vi "Final_Project_Follower_Template-1.vi"   [LabVIEW 2016]
uses:
  <vilib>/NXT/Block Support/NXT_InputPort.ctl
  <vilib>/NXT/Block Support/NXT_TimerIndex.ctl
  <vilib>/NXT/Block Support/NXT_OutputPort.ctl
  <vilib>/NXT/Dual Mode Library/Sensors/EV3_Color_Reflect.vi
  <vilib>/NXT/Dual Mode Library/Display/drawText_Right.vi
  <vilib>/NXT/NXTIO Xnodes/NXTIONodeSubVIs/NXTStopMotors.vi
  <vilib>/NXT/Dual Mode Library/Sensors/EV3_Ultrasonic_CM.vi
  <vilib>/NXT/NXTIO Xnodes/NXTIONodeSubVIs/NXTMoveMotors.vi
  <vilib>/NXT/Dual Mode Library/Display/drawNumber.vi
  <vilib>/NXT/Dual Mode Library/Display/drawNumber_float.vi
  <vilib>/NXT/Dual Mode Library/Display/drawText.vi
  <vilib>/NXT/Subs/LVHSConnector.ctl
  <vilib>/NXT/NXTIO Xnodes/AddressXNode/NXTIOAddress.xnode
  <vilib>/NXT/NXTIO Xnodes/NXTIOXNode/NXTIO.xnode
  <vilib>/NXT/LegoClasses/BrickReference/BrickReference.lvclass
types:
  T1 = typedef "LVHSConnector.ctl" = refnum<class "BrickReference.lvclass">
  T2 = typedef "NXT_InputPort.ctl" = u32
  T3 = typedef "NXT_TimerIndex.ctl" = u8
  T4 = typedef "NXT_OutputPort.ctl" = u8
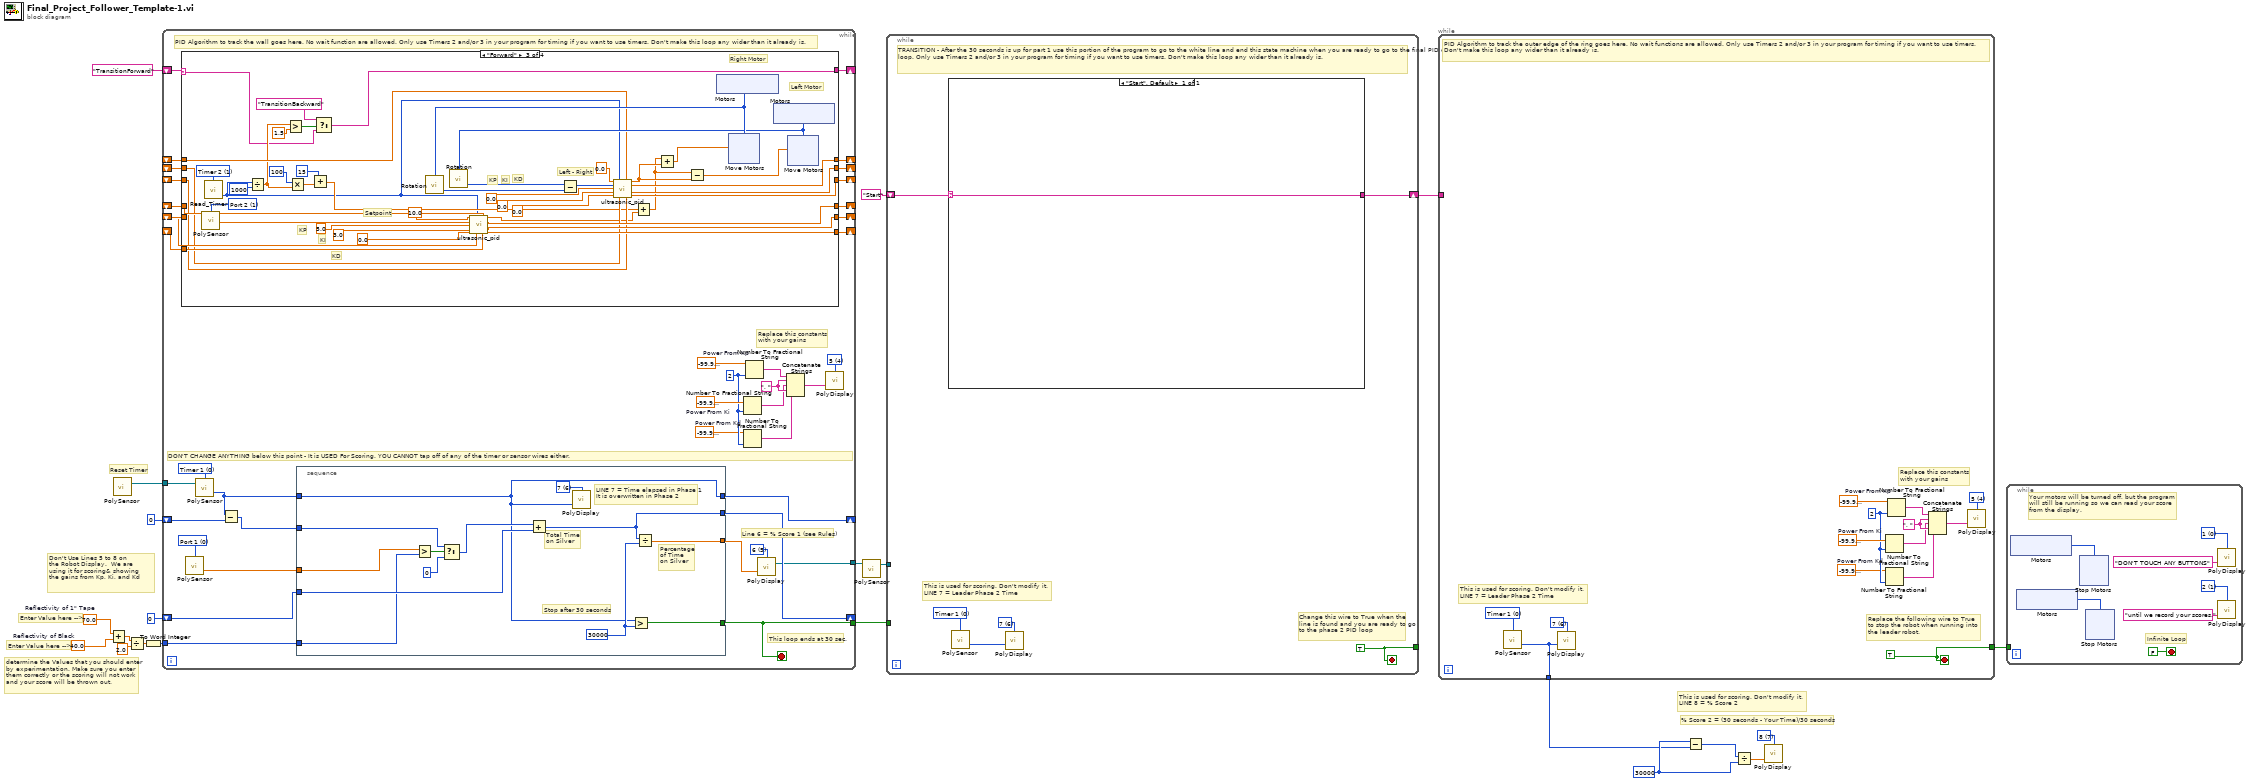
[diagram p0: block diagram]
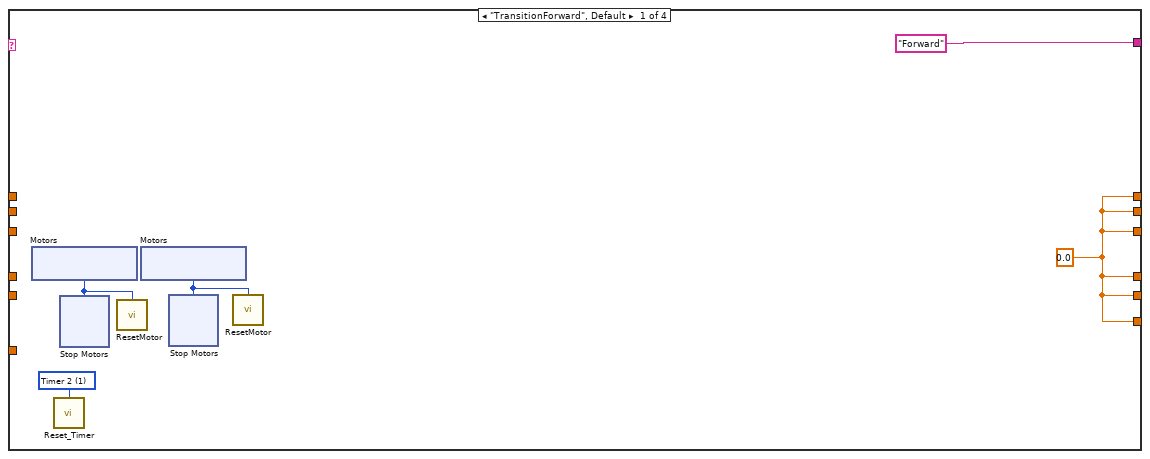
[diagram p2: hidden frame]
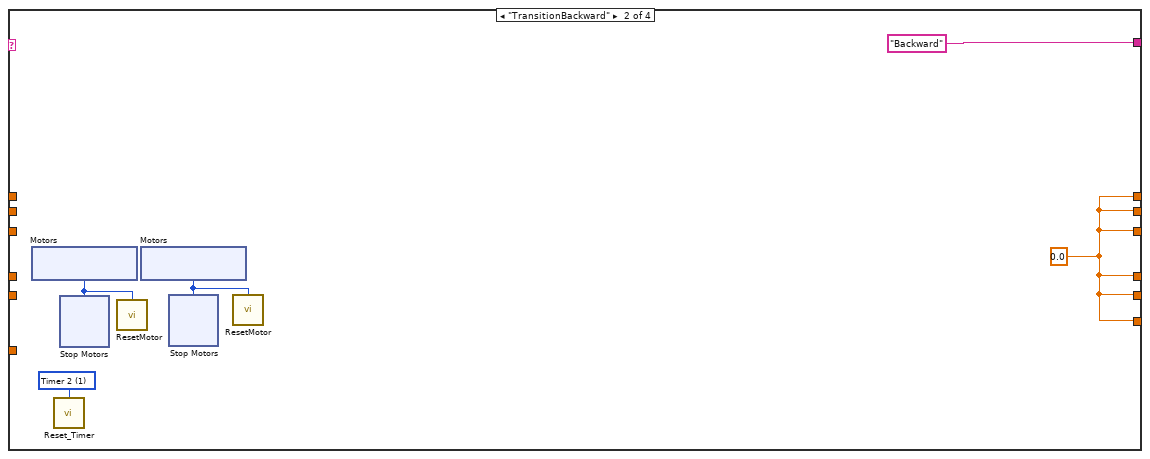
[diagram p3: hidden frame]
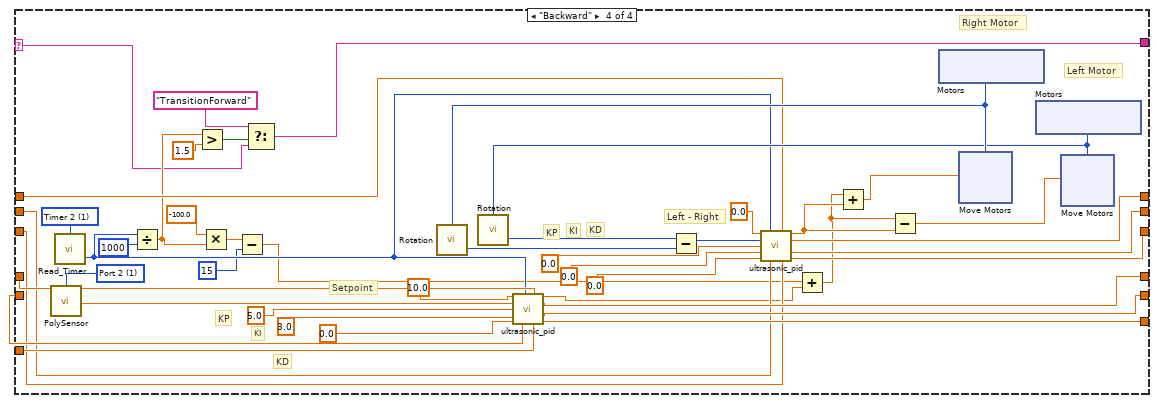
[diagram p4: hidden frame]
diagram:
  w5 = u32 30000 ("Value (msec)")
  w6 = i16 7 items=["1", "2", "3", "4", "5", "6", "7", "8", "9", "10", "11", "12"] ("Line")
  w12 = 40.0  # Reflectivity of Black
  w11 = 70.0  # Reflectivity of 1" Tape
  # "This is used for scoring. Don't modify it.\nLINE 8 = % Score 2"
  # "Don't Use Lines 5 to 8 on\nthe Robot Display.  We are \nusing it for scoring& showing \nthe gains from Kp, Ki, and Kd"
  # "% Score 2 = (30 seconds - Your Time)/30 seconds"
  # "Enter Value here -->"
  # "determine the Values that you should enter\nby experimentation. Make sure you enter \nthem correctly or the scoring will not work\nand your score will be thrown out."
  # "Enter Value here -->"
  # "Reset Timer"
  n1 = Add(x=w11, y=w12) -> (x+y=w10:dbl)
  n2 = call-poly <vilib>:"PolySensor.vi"() -> ("NXT/EV3"=w19:T1)  [unwired: 4 in]
  n3 = Divide(x=w10, y=2.0) -> (x/y=w9:dbl)
  n4 = To Word Integer(number=w9) -> (16bit integer=w16:i16)
  n5 = while {
    shift-right: [w56] -> _
    shift-left: i16 0 -> [w60]
    shift-right: [w57] -> _
    shift-left: i16 0 ("Value (msec)") -> [w59]
    tunnel: w19 -> [w55]
    tunnel: [w58] -> w18
    tunnel: w16 -> [w50]
    tunnel: [w46] -> w14
    shift-right: [w33] -> _
    shift-left: _ -> [w32]
    shift-right: [w34] -> _
    shift-left: _ -> [w31]
    shift-right: [w35] -> _
    shift-left: _ -> [w30]
    shift-right: [w29] -> _
    shift-left: _ -> [w26]
    shift-right: [w28] -> _
    shift-left: _ -> [w25]
    shift-right: [w27] -> _
    shift-left: _ -> [w24]
    shift-right: [w22] -> _
    shift-left: "TransitionForward" -> [w23]
    stop <- w58 stop-if-true
    w39 = ", " ("string")
    w42 = i16 2 ("precision (6)")
    w41 = sgl -99.9  # Power From Kd
    w43 = sgl -99.9  # Power From Ki
    w44 = sgl -99.9  # Power From Kp
    w45 = i16 4 items=["1", "2", "3", "4", "5", "6", "7", "8", "9", "10", "11", "12"] ("Line")
    w48 = i16 5 items=["1", "2", "3", "4", "5", "6", "7", "8", "9", "10", "11", "12"] ("Line")
    w52 = T2 0 items=["Port 1", "Port 2", "Port 3", "Port 4"] ("Port (Port 3)")
    w53 = T3 0 items=["Timer 1", "Timer 2", "Timer 3"] ("Timer (Timer 1)")
    # "Replace this constants\nwith your gains"
    # "DON'T CHANGE ANYTHING below this point - It is USED For Scoring. YOU CANNOT tap off of any of the timer or sensor wires either."
    # "Line 6 = % Score 1 (see Rules)"
    # "This loop ends at 30 sec."
    # "PID Algorithm to track the wall goes here. No wait function are allowed. Only use Timers 2 and/or 3 in your program for timing if you want to use timers. Don't make this loop any wider than it already is."
    n6 = case shown="\"Forward\"" w23 {
      selector: w23 -> [_ _ w97 w162]
      tunnel: [w61 w78 w137 w198] -> w35
      tunnel: [w61 w78 w136 w197] -> w34
      tunnel: [w61 w78 w135 w196] -> w33
      tunnel: w32 -> [_ _ w134 w195]
      tunnel: w31 -> [_ _ w133 w194]
      tunnel: w30 -> [_ _ w132 w193]
      tunnel: [w61 w78 w121 w182] -> w29
      tunnel: [w61 w78 w120 w181] -> w28
      tunnel: [w61 w78 w119 w180] -> w27
      tunnel: w26 -> [_ _ w114 w175]
      tunnel: w25 -> [_ _ w113 w174]
      tunnel: w24 -> [_ _ w112 w173]
      tunnel: ["Forward" ("t") "Backward" ("t") w95 w160] -> w22
      frame "TransitionForward", Default {
        w61 = sgl 0.0 ("Error")
        w65 = T3 1 items=["Timer 1", "Timer 2", "Timer 3"] ("Timer (Timer 1)")
        n7 = xnode "Motors"() -> ("Motor"=w64:T4)
        n8 = call <vilib>:"Reset_Timer.vi"("Timer (Timer 1)"=w65) -> ()  [unwired: 3 in, 1 out]
        n9 = xnode "Stop Motors"("Motors"=w64) -> ()  [unwired: 1 in, 1 out]
        n10 = call <vilib>:"ResetMotor.vi"("Port (All Ports)"=w64) -> ()  [unwired: 3 in, 1 out]
        n11 = xnode "Motors"() -> ("Motor"=w63:T4)
        n12 = xnode "Stop Motors"("Motors"=w63) -> ()  [unwired: 1 in, 1 out]
        n13 = call <vilib>:"ResetMotor.vi"("Port (All Ports)"=w63) -> ()  [unwired: 3 in, 1 out]
      }
      frame "TransitionBackward" {
        w78 = sgl 0.0 ("Error")
        w82 = T3 1 items=["Timer 1", "Timer 2", "Timer 3"] ("Timer (Timer 1)")
        n14 = xnode "Motors"() -> ("Motor"=w81:T4)
        n15 = call <vilib>:"Reset_Timer.vi"("Timer (Timer 1)"=w82) -> ()  [unwired: 3 in, 1 out]
        n16 = xnode "Stop Motors"("Motors"=w81) -> ()  [unwired: 1 in, 1 out]
        n17 = call <vilib>:"ResetMotor.vi"("Port (All Ports)"=w81) -> ()  [unwired: 3 in, 1 out]
        n18 = xnode "Motors"() -> ("Motor"=w80:T4)
        n19 = xnode "Stop Motors"("Motors"=w80) -> ()  [unwired: 1 in, 1 out]
        n20 = call <vilib>:"ResetMotor.vi"("Port (All Ports)"=w80) -> ()  [unwired: 3 in, 1 out]
      }
      frame "Forward" {
        w127 = T2 1 items=["Port 1", "Port 2", "Port 3", "Port 4"] ("Port (Port 1)")
        w139 = T3 1 items=["Timer 1", "Timer 2", "Timer 3"] ("Timer (Timer 1)")
        # "KD"
        # "KI"
        # "KP"
        # "Left - Right"
        # "Left Motor"
        # "Right Motor"
        # "KD"
        # "KP"
        # "KI"
        # "Setpoint"
        n21 = call-poly <vilib>:"PolySensor.vi"("Port (Port 1)"=w127) -> ("Centimeters"=w128:sgl)  [unwired: 2 in, 1 out]
        n22 = call <vilib>:"Read_Timer.vi"("Timer (Timer 1)"=w139) -> ("Value (msec)"=w102:u32)  [unwired: 2 in, 1 out]
        n23 = Divide(x=w102, y=u32 1000) -> (x/y=w100:dbl)
        n24 = Greater?(x=w100, y=1.5) -> (0:w98:bool)
        n25 = Multiply(x=u32 100, y=w100) -> (x*y=w107:dbl)
        n26 = Add(x=u32 15, y=w107) -> (x+y=w103:dbl)
        n27 = Select(t="TransitionBackward", s=w98, f=w97) -> (s? t:f=w95:string)
        n28 = call "ultrasonic_pid.vi"("Setpoint"=sgl 10.0, "Time"=w102, "Error"=w132, "Input"=w128, "KP"=sgl 5.0, "KI"=3.0, "KD"=0.0, "Previous Time"=w133, "Accumulated Error"=w134) -> ("Output"=w105:dbl, "Error"=w137:sgl, "Current Time"=w136:dbl, "Accumulated Error"=w135:dbl)  [unwired: 3 in]
        n29 = Add(x=w103, y=w105) -> (x+y=w104:dbl)
        n30 = xnode "Motors"() -> ("Motor"=w126:T4)
        n31 = call <vilib>:"Rotation.vi"("Port (Port A)"=w126) -> ("Angle of Rotation"=w124:i32)  [unwired: 2 in, 1 out]
        n32 = xnode "Motors"() -> ("Motor"=w125:T4)
        n33 = call <vilib>:"Rotation.vi"("Port (Port A)"=w125) -> ("Angle of Rotation"=w123:i32)  [unwired: 2 in, 1 out]
        n34 = Subtract(x=w123, y=w124) -> (x-y=w122:i32)
        n35 = call "ultrasonic_pid.vi"("Setpoint"=sgl 0.0, "Time"=w102, "Error"=w112, "Input"=w122, "KP"=sgl 0.0, "KI"=0.0, "KD"=0.0, "Previous Time"=w113, "Accumulated Error"=w114) -> ("Output"=w111:dbl, "Error"=w119:sgl, "Current Time"=w120:dbl, "Accumulated Error"=w121:dbl)  [unwired: 3 in]
        n36 = Add(x=w104, y=w111) -> (x+y=w110:dbl)
        n37 = Subtract(x=w104, y=w111) -> (x-y=w109:dbl)
        n38 = xnode "Move Motors"("Power/Speed 1"=w110, "Motors"=w126) -> ()  [unwired: 1 in, 1 out]
        n39 = xnode "Move Motors"("Power/Speed 1"=w109, "Motors"=w125) -> ()  [unwired: 1 in, 1 out]
      }
      frame "Backward" {
        w188 = T2 1 items=["Port 1", "Port 2", "Port 3", "Port 4"] ("Port (Port 1)")
        w200 = T3 1 items=["Timer 1", "Timer 2", "Timer 3"] ("Timer (Timer 1)")
        # "KD"
        # "KI"
        # "KP"
        # "Left - Right"
        # "Left Motor"
        # "Right Motor"
        # "KD"
        # "KP"
        # "KI"
        # "Setpoint"
        n40 = call-poly <vilib>:"PolySensor.vi"("Port (Port 1)"=w188) -> ("Centimeters"=w189:sgl)  [unwired: 2 in, 1 out]
        n41 = call <vilib>:"Read_Timer.vi"("Timer (Timer 1)"=w200) -> ("Value (msec)"=w167:u32)  [unwired: 2 in, 1 out]
        n42 = Divide(x=w167, y=u32 1000) -> (x/y=w165:dbl)
        n43 = Greater?(x=w165, y=1.5) -> (0:w163:bool)
        n44 = Multiply(x=-100.0, y=w165) -> (x*y=w158:dbl)
        n45 = Subtract(x=w158, y=u32 15 ("x")) -> (x-y=w156:dbl)
        n46 = Select(t="TransitionForward", s=w163, f=w162) -> (s? t:f=w160:string)
        n47 = call "ultrasonic_pid.vi"("Setpoint"=sgl 10.0, "Time"=w167, "Error"=w193, "Input"=w189, "KP"=sgl 5.0, "KI"=3.0, "KD"=0.0, "Previous Time"=w194, "Accumulated Error"=w195) -> ("Output"=w169:dbl, "Error"=w198:sgl, "Current Time"=w197:dbl, "Accumulated Error"=w196:dbl)  [unwired: 3 in]
        n48 = Add(x=w156, y=w169) -> (x+y=w168:dbl)
        n49 = xnode "Motors"() -> ("Motor"=w187:T4)
        n50 = call <vilib>:"Rotation.vi"("Port (Port A)"=w187) -> ("Angle of Rotation"=w185:i32)  [unwired: 2 in, 1 out]
        n51 = xnode "Motors"() -> ("Motor"=w186:T4)
        n52 = call <vilib>:"Rotation.vi"("Port (Port A)"=w186) -> ("Angle of Rotation"=w184:i32)  [unwired: 2 in, 1 out]
        n53 = Subtract(x=w184, y=w185) -> (x-y=w183:i32)
        n54 = call "ultrasonic_pid.vi"("Setpoint"=sgl 0.0, "Time"=w167, "Error"=w173, "Input"=w183, "KP"=sgl 0.0, "KI"=0.0, "KD"=0.0, "Previous Time"=w174, "Accumulated Error"=w175) -> ("Output"=w172:dbl, "Error"=w180:sgl, "Current Time"=w181:dbl, "Accumulated Error"=w182:dbl)  [unwired: 3 in]
        n55 = Add(x=w168, y=w172) -> (x+y=w171:dbl)
        n56 = Subtract(x=w168, y=w172) -> (x-y=w170:dbl)
        n57 = xnode "Move Motors"("Power/Speed 1"=w171, "Motors"=w187) -> ()  [unwired: 1 in, 1 out]
        n58 = xnode "Move Motors"("Power/Speed 1"=w170, "Motors"=w186) -> ()  [unwired: 1 in, 1 out]
      }
    }
    n59 = call-poly <vilib>:"PolySensor.vi"("Port (Port 1)"=w52) -> ("Scaled Value"=w51:sgl)  [unwired: 2 in, 1 out]
    n60 = call-poly <vilib>:"PolySensor.vi"("NXT/EV3"=w55, "Timer (Timer 1)"=w53) -> ("Value (msec)"=w54:u32)  [unwired: 1 in, 1 out]
    n61 = Subtract(x=w54, y=w59) -> (x-y=w49:u32)
    n62 = stacked-sequence {
      tunnel: w60 -> [w229]
      tunnel: [w219] -> w47
      tunnel: w54 -> [w217]
      tunnel: [w228] -> w58
      tunnel: w51 -> [w223]
      tunnel: w49 -> [w225]
      tunnel: [w217] -> w57
      tunnel: [w221] -> w56
      tunnel: w50 -> [w222]
      frame #0 {
        w218 = i16 6 items=["1", "2", "3", "4", "5", "6", "7", "8", "9", "10", "11", "12"] ("Line")
        w220 = u32 30000 ("Value (msec)")
        # "LINE 7 = Time elapsed in Phase 1\nIt is overwritten in Phase 2"
        # "Percentage\nof Time\non Silver"
        # "Stop after 30 seconds"
        # "Total Time\non Silver"
        n63 = Greater?(x=w223, y=w222) -> (0:w226:bool)
        n64 = Select(t=w225, s=w226, f=i16 0) -> (s? t:f=w224:u32)
        n65 = Add(x=w224, y=w229) -> (x+y=w221:u32)
        n66 = call-poly <vilib>:"PolyDisplay.vi"("number"=w217, "Line"=w218) -> ()  [unwired: 2 in, 1 out]
        n67 = Greater?(x=w217, y=w220) -> (0:w228:bool)
        n68 = Divide(x=w221, y=w220) -> (x/y=w219:dbl)
      }
    }
    n69 = Number To Fractional String(number=w43, precision (6)=w42) -> (F-format string=w38:string)  [unwired: 2 in]
    n70 = Number To Fractional String(number=w41, precision (6)=w42) -> (F-format string=w37:string)  [unwired: 2 in]
    n71 = Number To Fractional String(number=w44, precision (6)=w42) -> (F-format string=w40:string)  [unwired: 2 in]
    n72 = call-poly <vilib>:"PolyDisplay.vi"("number"=w47, "Line"=w48) -> ("NXT/EV3"=w46:T1)  [unwired: 2 in]
    n73 = Concatenate Strings(w40, w39, w38, w39, w37) -> (w36:string)
    n74 = call-poly <vilib>:"PolyDisplay.vi"("Text"=w36, "Line"=w45) -> ()  [unwired: 2 in, 1 out]
  }
  n75 = call-poly <vilib>:"PolySensor.vi"("NXT/EV3"=w14) -> ("NXT/EV3"=w13:T1)  [unwired: 3 in]
  n76 = while {
    tunnel: w18 -> [_]
    shift-right: [w234] -> w7
    shift-left: "Start" -> [w235]
    tunnel: w13 -> [_]
    tunnel: [w230] -> _
    stop <- w230 stop-if-true
    w230 = TRUE
    w231 = i16 6 items=["1", "2", "3", "4", "5", "6", "7", "8", "9", "10", "11", "12"] ("Line")
    w233 = T3 0 items=["Timer 1", "Timer 2", "Timer 3"] ("Timer (Timer 1)")
    # "This is used for scoring. Don't modify it.\nLINE 7 = Leader Phase 2 Time"
    # "Change this wire to True when the line is found and you are ready to go to the phase 2 PID loop"
    # "TRANSITION - After the 30 seconds is up for part 1 use this portion of the program to go to the white line and end this state machine when you are ready to go to the final PID control loop. Only use Timers 2 and/or 3 in your program for timing if you want to use timers. Don't make this loop any wider than it already is."
    n77 = case shown="\"Start\", Default" w235 {
      selector: w235 -> [w236]
      tunnel: [w236] -> w234
      frame "Start", Default {
      }
    }
    n78 = call-poly <vilib>:"PolySensor.vi"("Timer (Timer 1)"=w233) -> ("Value (msec)"=w232:u32)  [unwired: 2 in, 1 out]
    n79 = call-poly <vilib>:"PolyDisplay.vi"("number"=w232, "Line"=w231) -> ()  [unwired: 2 in, 1 out]
  }
  n80 = while {
    tunnel: [w248] -> w8
    tunnel: w7 -> [_]
    tunnel: [w247] -> w4
    stop <- w248 stop-if-true
    w240 = ", " ("string")
    w243 = i16 2 ("precision (6)")
    w242 = sgl -99.9  # Power From Kd
    w244 = sgl -99.9  # Power From Ki
    w245 = sgl -99.9  # Power From Kp
    w246 = i16 4 items=["1", "2", "3", "4", "5", "6", "7", "8", "9", "10", "11", "12"] ("Line")
    w248 = TRUE
    w249 = i16 6 items=["1", "2", "3", "4", "5", "6", "7", "8", "9", "10", "11", "12"] ("Line")
    w250 = T3 0 items=["Timer 1", "Timer 2", "Timer 3"] ("Timer (Timer 1)")
    # "Replace this constants\nwith your gains"
    # "This is used for scoring. Don't modify it.\nLINE 7 = Leader Phase 2 Time"
    # "PID Algorithm to track the outer edge of the ring goes here. No wait functions are allowed. Only use Timers 2 and/or 3 in your program for timing if you want to use timers.\nDon't make this loop any wider than it already is."
    # "Replace the following wire to True\nto stop the robot when running into \nthe leader robot."
    n81 = call-poly <vilib>:"PolySensor.vi"("Timer (Timer 1)"=w250) -> ("Value (msec)"=w247:u32)  [unwired: 2 in, 1 out]
    n82 = call-poly <vilib>:"PolyDisplay.vi"("number"=w247, "Line"=w249) -> ()  [unwired: 2 in, 1 out]
    n83 = Number To Fractional String(number=w244, precision (6)=w243) -> (F-format string=w239:string)  [unwired: 2 in]
    n84 = Number To Fractional String(number=w242, precision (6)=w243) -> (F-format string=w238:string)  [unwired: 2 in]
    n85 = Number To Fractional String(number=w245, precision (6)=w243) -> (F-format string=w241:string)  [unwired: 2 in]
    n86 = Concatenate Strings(w241, w240, w239, w240, w238) -> (w237:string)
    n87 = call-poly <vilib>:"PolyDisplay.vi"("Text"=w237, "Line"=w246) -> ()  [unwired: 2 in, 1 out]
  }
  n88 = Subtract(x=w5, y=w4) -> (x-y=w3:u32)
  n89 = Divide(x=w3, y=w5) -> (x/y=w2:dbl)
  n90 = call-poly <vilib>:"PolyDisplay.vi"("number"=w2, "Line"=w6) -> ()  [unwired: 2 in, 1 out]
  n91 = while {
    tunnel: w8 -> [_]
    stop <- FALSE stop-if-true
    w251 = i16 1 items=["1", "2", "3", "4", "5", "6", "7", "8", "9", "10", "11", "12"] ("Line")
    w254 = i16 0 items=["1", "2", "3", "4", "5", "6", "7", "8", "9", "10", "11", "12"] ("Line")
    # "Your motors will be turned off, but the program\nwill still be running so we can read your score\nfrom the display."
    # "Infinite Loop"
    n92 = xnode "Motors"() -> ("Motor"=w256:T4)
    n93 = xnode "Motors"() -> ("Motor"=w255:T4)
    n94 = xnode "Stop Motors"("Motors"=w256) -> ()  [unwired: 1 in, 1 out]
    n95 = xnode "Stop Motors"("Motors"=w255) -> ()  [unwired: 1 in, 1 out]
    n96 = call-poly <vilib>:"PolyDisplay.vi"("Text"="DON'T TOUCH ANY BUTTONS", "Line"=w254) -> ()  [unwired: 2 in, 1 out]
    n97 = call-poly <vilib>:"PolyDisplay.vi"("Text"="until we record your scores.", "Line"=w251) -> ()  [unwired: 2 in, 1 out]
  }
